vi "STEPkgDriver_LINC_Client.vi"() -> ()   [LabVIEW 2018, in "STEPkgDriver_LINC.lvlib"]
uses:
  STEPkgDriver_LINC.lvlib
  LINC/LINC.lvclass
  LINC/LINC Server Telemetry Prototype.ctl
  LINC/LINC Client Housekeeping.ctl
panel:
  in  "Address:":string="localhost"
  out "connected":bool
  in  "SET_U8_SCALED":dbl
  out "TEST_PACKET":T1={"COUNTER"=0, "NUMBER"=0.0, "STRING"="0000000000", "BOOLEAN"=FALSE, "ENUM"=enum."ENUM_ONE", "RING"=0, "ARRAY_U32"=[], "U8_SCALED"=0} {"U8_SCALED" format="%.3f"; "RING" items=["RING_ONE"=0, "RING_TWO"=1, "RING_THREE"=2, "RING_FOUR"=4]}
  in  "SET_ARRAY_U32":u32[](array[numeric])
  out "TELEMETRY:":string
  in  "SET_ERROR":bool
  in  "ERROR":errorcluster
  in  "SET_RING":u16(ring) items=["RING_ONE"=0, "RING_TWO"=1, "RING_THREE"=2, "RING_FOUR"=4]
  in  "SET_ENUM":enum16{"ENUM_ONE", "ENUM_TWO", "ENUM_THREE"}(ring)
  in  "SET_BOOLEAN":bool
  in  "SET_ALL":bool
  in  "SET_ALL":T2 {"RING" items=["RING_ONE"=0, "RING_TWO"=1, "RING_THREE"=2, "RING_FOUR"=4]}
  in  "SET_STRING":string
  in  "SET_NUMBER":dbl
  in  "COUNTER_INC":bool
  in  "COUNTER_RESET":bool
  in  "Port:":u16=8000 min=1025 step=1
  in  "close":bool
  # "Manual Commands:"
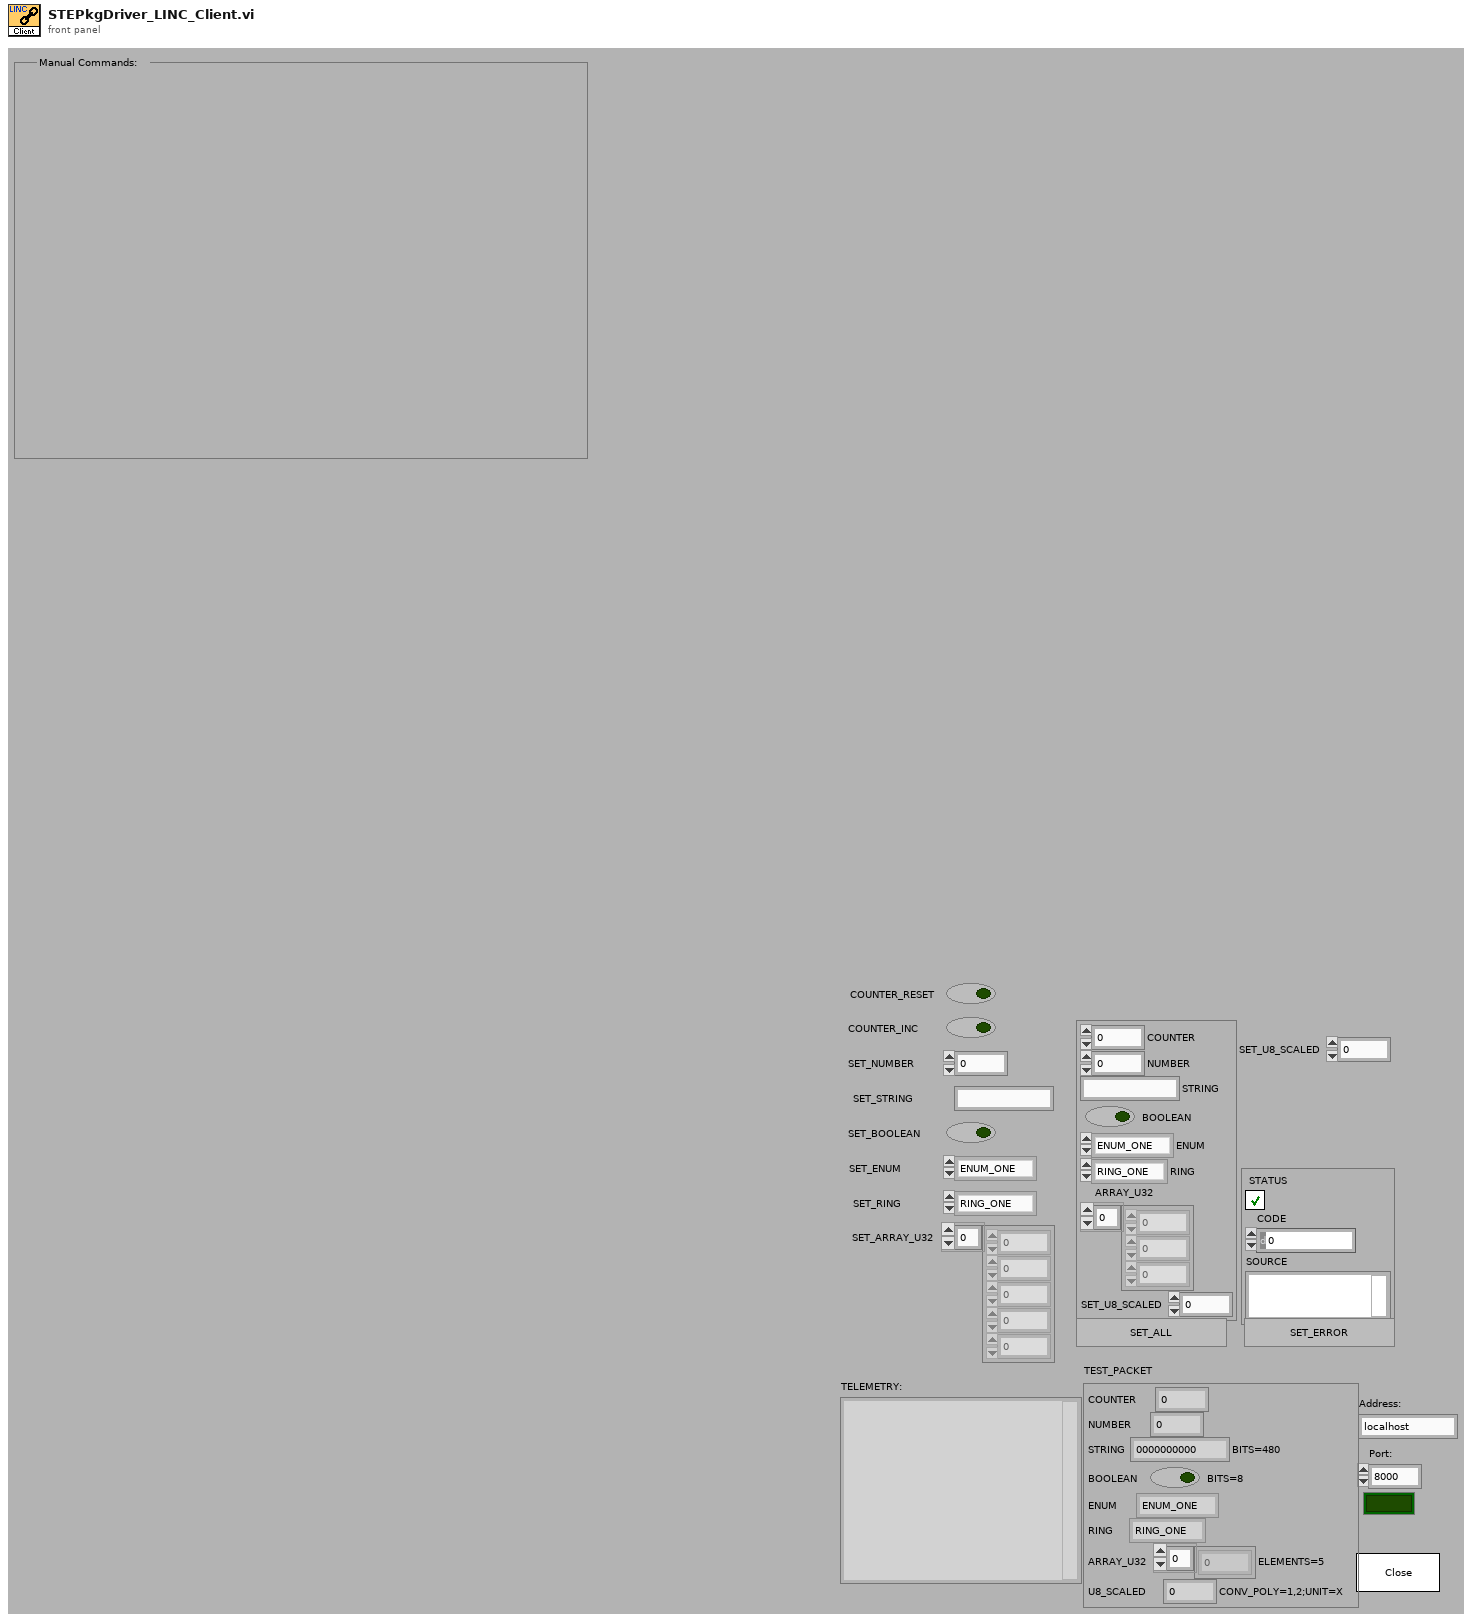
[diagram p1: front panel]
types:
  T1 = typedef "STEPkgDriver_LINC.lvlib/LINC Server Telemetry Prototype.ctl" = cluster{"COUNTER":u32, "NUMBER":dbl, "STRING":string, "BOOLEAN":bool, "ENUM":enum8{"ENUM_ONE", "ENUM_TWO", "ENUM_THREE"}, "RING":u8, "ARRAY_U32":u32[], "U8_SCALED":u8}
  T2 = cluster{"COUNTER":u32, "NUMBER":dbl, "STRING":string, "BOOLEAN":bool, "ENUM":enum16{"ENUM_ONE", "ENUM_TWO", "ENUM_THREE"}, "RING":u16, "ARRAY_U32":u32[], "SET_U8_SCALED":u8}
  T3 = typedef "STEPkgDriver_LINC.lvlib/LINC Client Housekeeping.ctl" = cluster{"TEST_PACKET":T1}
  T4 = cluster{"binary value (F)":bool, "include unit (F)":bool}
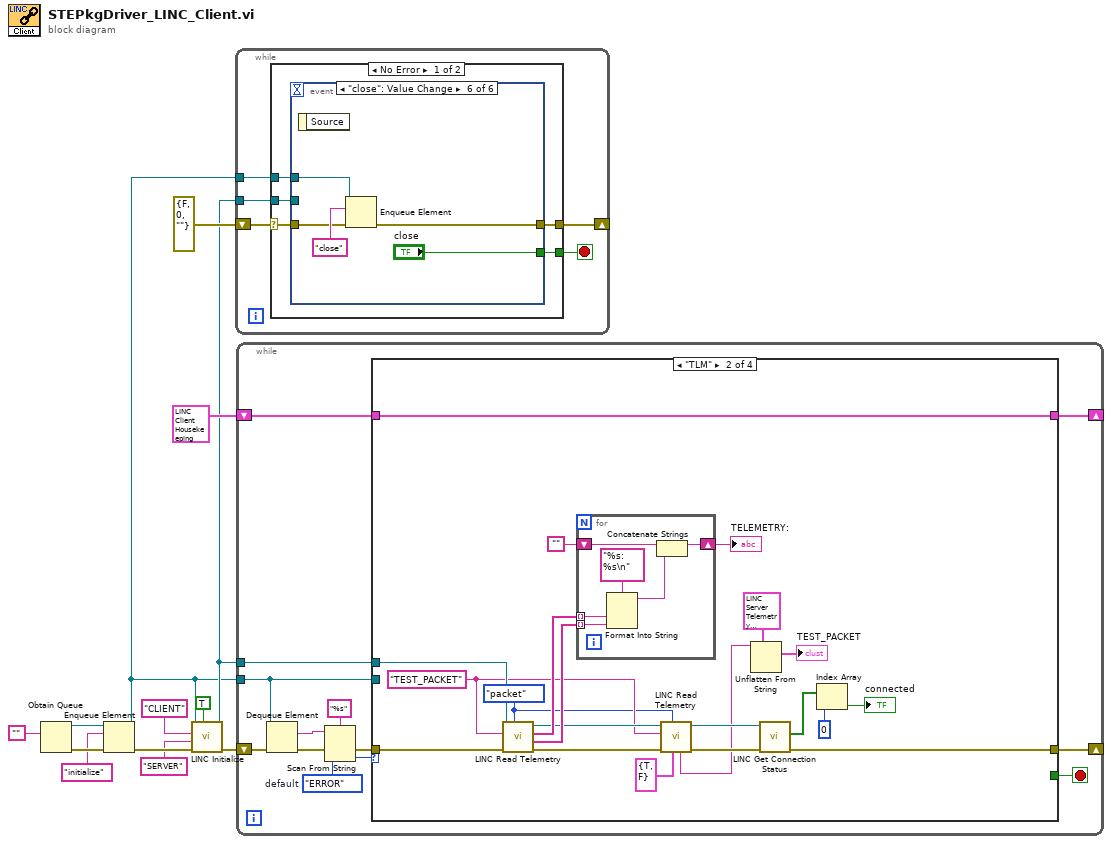
[diagram p0: block diagram]
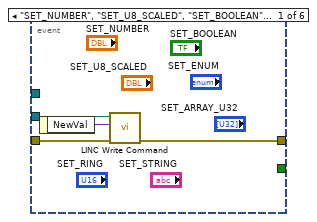
[diagram p2: hidden frame]
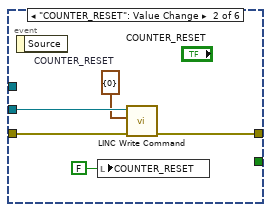
[diagram p3: hidden frame]
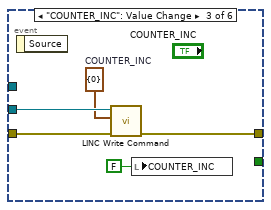
[diagram p4: hidden frame]
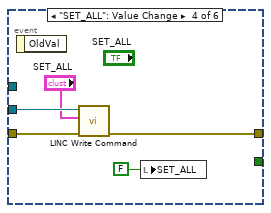
[diagram p5: hidden frame]
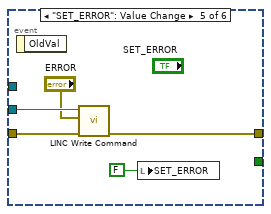
[diagram p6: hidden frame]
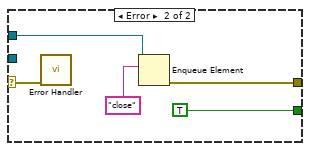
[diagram p7: hidden frame]
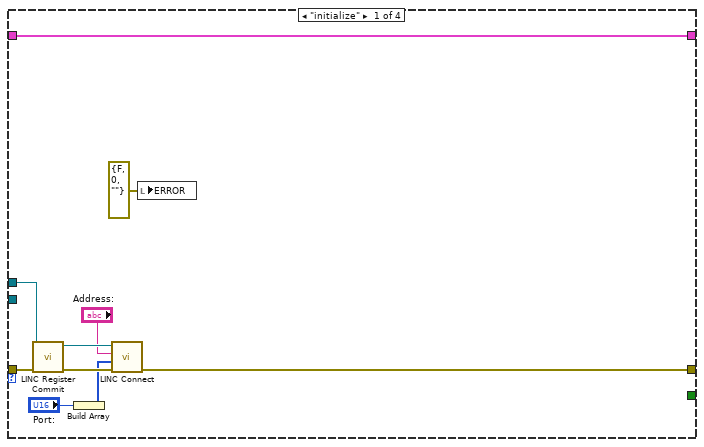
[diagram p8: hidden frame]
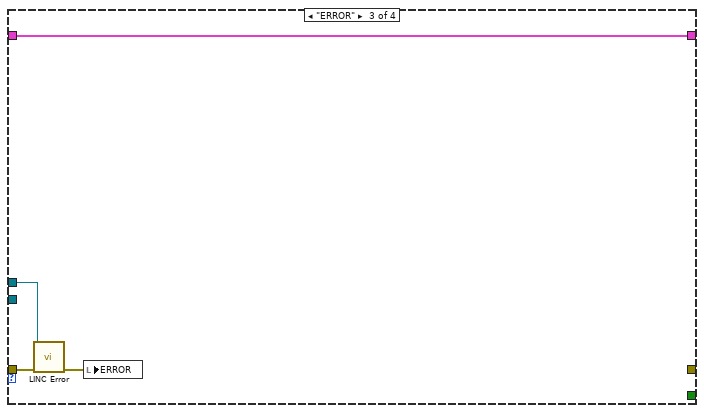
[diagram p9: hidden frame]
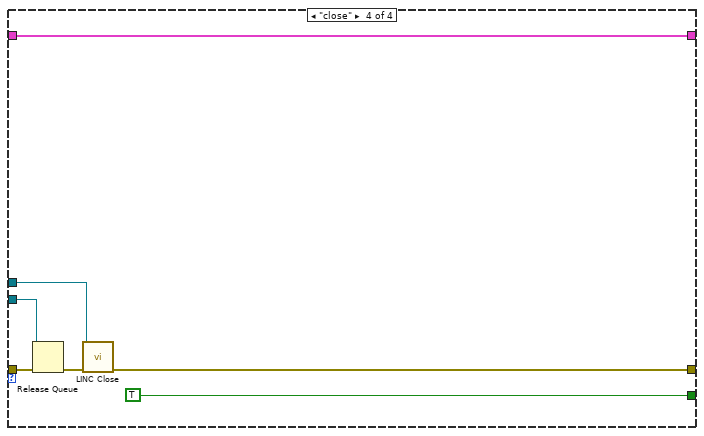
[diagram p10: hidden frame]
diagram:
  n1 = Obtain Queue(element data type="") -> (queue out=w11:refnum<queue>, error out=w12:errorcluster)  [unwired: 3 in, 2 out]
  n2 = Enqueue Element(queue=w11, element="initialize", error in (no error)=w12) -> (queue out=w3:refnum<queue>, error out=w9:errorcluster)  [unwired: 1 in, 1 out]
  n3 = call "LINC Initialize.vi"("client session (F)"=TRUE, "error in (no error)"=w9, "server name (\"\")"="SERVER" ("server name (\"\")"), "target name"="CLIENT", "application queue"=w3) -> ("error out"=w7:errorcluster, "LINC session"=w5:refnum<class "LINC.lvclass">)  [unwired: 1 in, 4 out]
  n4 = while {
    shift-right: [w16] -> _
    shift-left: errorcluster {"status"=FALSE, "code"=0, "source"=""} ("error out") -> [w18]
    tunnel: w5 -> [w15]
    tunnel: w3 -> [w14]
    stop <- w17 stop-if-true
    n5 = case shown="No Error" w18 {
      selector: w18 -> [w22 w56]
      tunnel: [w21 TRUE] -> w17
      tunnel: [w23 w53] -> w16
      tunnel: w15 -> [w20 _]
      tunnel: w14 -> [w19 w54]
      frame No Error {
        n6 = event shown="[5] \"close\": Value Change" {
          selector: _ -> [_ _ _ _ _ _]
          dyn-events: _ -> [_ _ _ _ _ _]
          timeout: _ -> [_ _ _ _ _ _]
          tunnel: [w26 w31 w36 w41 w46 w49] -> w23
          tunnel: w22 -> [w27 w32 w37 w42 w47 w50]
          tunnel: [_ _ _ _ _ "close"] -> w21
          tunnel: w20 -> [w25 w30 w35 w40 w45 _]
          tunnel: w19 -> [_ _ _ _ _ w48]
          event "SET_NUMBER", "SET_U8_SCALED", "SET_BOOLEAN", "SET_RING", "SET_ENUM", "SET_STRING", "SET_ARRAY_U32": Value Change {
            n7 = event-data() -> ("NewVal"=w24:variant)  [unwired: 1 out]
            n8 = call "LINC Write Command.vi"("error in (no error)"=w27, "packet"=w24, "LINC session"=w25) -> ("error out"=w26:errorcluster)  [unwired: 5 in, 3 out]
          }
          event "COUNTER_RESET": Value Change {
            w29 = cluster{"DUMMY":u8} {"DUMMY"=0}  # COUNTER_RESET
            n9 = event-data() -> ()  [unwired: 2 out]
            n10 = local write "COUNTER_RESET"(FALSE ("COUNTER_RESET")) -> ()
            n11 = call "LINC Write Command.vi"("error in (no error)"=w32, "packet"=w29, "LINC session"=w30) -> ("error out"=w31:errorcluster)  [unwired: 5 in, 3 out]
          }
          event "COUNTER_INC": Value Change {
            w34 = cluster{"DUMMY":u8} {"DUMMY"=0}  # COUNTER_INC
            n12 = event-data() -> ()  [unwired: 2 out]
            n13 = call "LINC Write Command.vi"("error in (no error)"=w37, "packet"=w34, "LINC session"=w35) -> ("error out"=w36:errorcluster)  [unwired: 5 in, 3 out]
            n14 = local write "COUNTER_INC"(FALSE ("COUNTER_INC")) -> ()
          }
          event "SET_ALL": Value Change {
            n15 = event-data() -> ()  [unwired: 2 out]
            n16 = call "LINC Write Command.vi"("error in (no error)"=w42, "packet"="SET_ALL", "LINC session"=w40) -> ("error out"=w41:errorcluster)  [unwired: 5 in, 3 out]
            n17 = local write "SET_ALL"(FALSE ("SET_ALL")) -> ()
          }
          event "SET_ERROR": Value Change {
            n18 = event-data() -> ()  [unwired: 2 out]
            n19 = call "LINC Write Command.vi"("error in (no error)"=w47, "packet"="ERROR", "LINC session"=w45) -> ("error out"=w46:errorcluster)  [unwired: 5 in, 3 out]
            n20 = local write "SET_ERROR"(FALSE ("SET_ERROR")) -> ()
          }
          event "close": Value Change {
            n21 = event-data() -> ()  [unwired: 2 out]
            n22 = Enqueue Element(queue=w48, element="close", error in (no error)=w50) -> (error out=w49:errorcluster)  [unwired: 1 in, 2 out]
          }
        }
      }
      frame Error {
        n23 = call "Error Handler.vi"("error in (no error)"=w56) -> ()  [unwired: 9 in, 2 out]
        n24 = Enqueue Element(queue=w54, element="close") -> (error out=w53:errorcluster)  [unwired: 2 in, 2 out]
      }
    }
  }
  n25 = while {
    shift-left: w7 -> [w63]
    shift-right: [w70] -> _
    tunnel: w3 -> [w62]
    shift-right: [w60] -> _
    shift-left: T3 {"TEST_PACKET"={"COUNTER"=0, "NUMBER"=0.0, "STRING"="", "BOOLEAN"=FALSE, "ENUM"=enum."ENUM_ONE", "RING"=0, "ARRAY_U32"=[], "U8_SCALED"=0}} -> [w61]
    tunnel: w5 -> [w58]
    stop <- w64 stop-if-true
    w66 = enum16{"initialize", "TLM", "ERROR", "close"}."ERROR"  # default
    n26 = Dequeue Element(queue=w62, error in (no error)=w63) -> (element=w59:string, error out=w68:errorcluster)  [unwired: 1 in, 2 out]
    n27 = Scan From String(format string="%s", input string=w59, error in=w68, default 1=w66) -> (error out=w67:errorcluster, output 1=w65:enum16{"initialize", "TLM", "ERROR", "close"})  [unwired: 1 in, 2 out]
    n28 = case shown="\"TLM\"" w65 {
      tunnel: w67 -> [w78 w96 w110 w116]
      tunnel: [w72 w94 _ w112] -> w70
      tunnel: [_ _ _ TRUE] -> w64
      tunnel: w62 -> [_ _ _ w117]
      tunnel: w61 -> [w73 w101 w111 w115]
      tunnel: [w73 w101 w111 w115] -> w60
      tunnel: w58 -> [w77 w95 w108 w113]
      frame "initialize" {
        n29 = call "LINC Register Commit.vi"("error in (no error)"=w78, "LINC session"=w77) -> ("error out"=w80:errorcluster, "dup LINC session"=w79:refnum<class "LINC.lvclass">)  [unwired: 1 in, 7 out]
        n30 = Build Array("Port:") -> (w74:u16[])
        n31 = call "LINC Connect.vi"("error in (no error)"=w80, "ports"=w74, "address"="Address:", "LINC session"=w79) -> ("error out"=w72:errorcluster)  [unwired: 6 in, 1 out]
        n32 = local write "ERROR"(errorcluster {"STATUS"=FALSE, "CODE"=0, "SOURCE"=""} ("ERROR")) -> ()
      }
      frame "TLM" {
        w82 = "TEST_PACKET" ("packet name")
        w81 = enum16{"single", "packet", "all"}."packet" ("mode (single)")
        n33 = call "LINC Read Telemetry.vi"("mode (single)"=w81, "error in (no error)"=w96, "packet name"=w82, "LINC session"=w95) -> ("error out"=w90:errorcluster, "item values"=w99:string[], "item names"=w100:string[], "dup LINC session"=w89:refnum<class "LINC.lvclass">)  [unwired: 3 in, 1 out]
        n34 = for {
          tunnel: w100 -> [w107] mode=indexing
          tunnel: w99 -> [w106] mode=indexing
          shift-right: [w102] -> w97
          shift-left: "" -> [w104]
          n35 = Format Into String(format string="%s: %s\n", w107, w106) -> (resulting string=w103:string)  [unwired: 2 in, 1 out]
          n36 = Concatenate Strings(w104, w103) -> (w102:string)
        }
        "TELEMETRY:" <- w97
        n37 = call "LINC Read Telemetry.vi"("options"=T4 {"binary value (F)"=TRUE, "include unit (F)"=FALSE}, "mode (single)"=w81, "error in (no error)"=w90, "packet name"=w82, "LINC session"=w89) -> ("error out"=w88:errorcluster, "dup LINC session"=w87:refnum<class "LINC.lvclass">, "flattened data"=w85:string)  [unwired: 2 in, 2 out]
        n38 = Unflatten From String(type=T1 {"COUNTER"=0, "NUMBER"=0.0, "STRING"="0000000000", "BOOLEAN"=FALSE, "ENUM"=enum."ENUM_ONE", "RING"=0, "ARRAY_U32"=[], "U8_SCALED"=0} ("TEST_PACKET"), binary string=w85) -> (value=→"TEST_PACKET":T1)  [unwired: 3 in, 2 out]
        n39 = call "LINC Get Connection Status.vi"("error in (no error)"=w88, "LINC session"=w87) -> ("error out"=w94:errorcluster, "connected"=w93:bool[])  [unwired: 7 in, 1 out]
        n40 = Index Array(array=w93, index=0) -> (element=→"connected":bool)
      }
      frame "ERROR" {
        n41 = call "LINC Error.vi"("error in (no error)"=w110, "LINC session"=w108) -> ("error out"=w109:errorcluster)  [unwired: 8 in, 1 out]
        n42 = local write "ERROR"(w109) -> ()
      }
      frame "close" {
        n43 = Release Queue(queue=w117, error in (no error)=w116) -> (error out=w114:errorcluster)  [unwired: 3 out]
        n44 = call "LINC Close.vi"("error in (no error)"=w114, "LINC session"=w113) -> ("error out"=w112:errorcluster)  [unwired: 9 out]
      }
    }
  }
